vi "OT-PSD for stage.vi"() -> ()   [LabVIEW 2014]
uses:
  <vilib>/Analysis/2dsp.llb/Real FFT.vi
  <vilib>/Analysis/8numeric.llb/1D Numeric Integration.vi
  <vilib>/Utility/file.llb/Read From Spreadsheet File (DBL).vi
  <vilib>/Analysis/NI_AALPro.lvlib
  <vilib>/Analysis/NI_AALBase.lvlib
panel:
  out "variance":dbl format="%0.2f"
  out "standard deviation":dbl format="%0.2f"
  out "frequency":dbl[](array[numeric])
  out "Integrated freq":dbl[](array[numeric])
  out "df":dbl
  in  "sampling frequency (Hz)":i32
  in  "Tab Control":T1(tab)
  out "XY Graph":cluster{dbl[], "Filtered X":dbl[]}(graph)
  out "PSD 4":cluster{dbl[], dbl[]}(graph)
  out "PSD":cluster{dbl[], dbl[]}(graph)
  out "AutoPSD 2":cluster{dbl[], dbl[]}(graph)
  out "AutoPSD":cluster{dbl[], dbl[]}(graph)
  out "PSD 3":cluster{dbl[], dbl[]}(graph)
  out "PSD 2":cluster{dbl[], dbl[]}(graph)
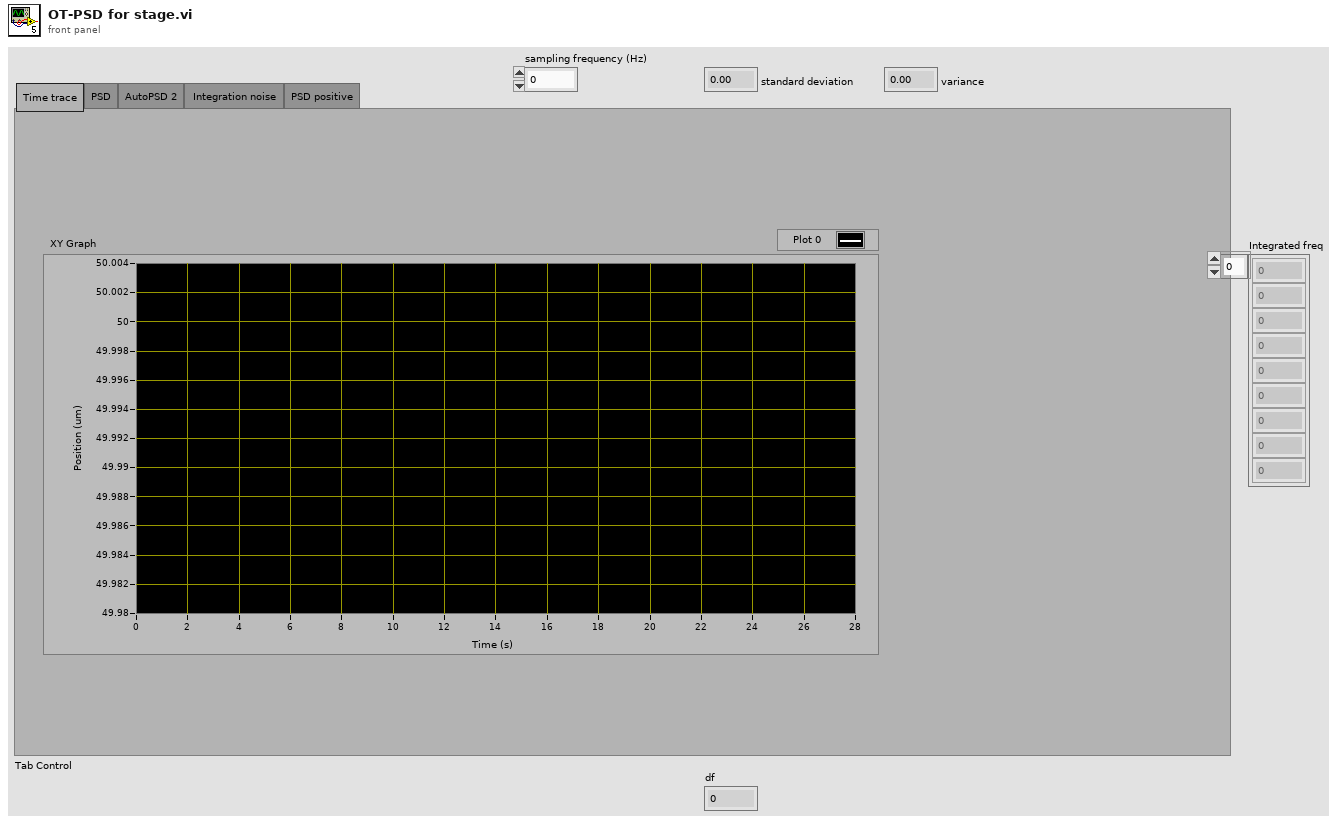
[diagram p1: front panel]
types:
  T1 = enum32{"Time trace", "PSD", "AutoPSD 2", "Integration noise ", "PSD positive"}
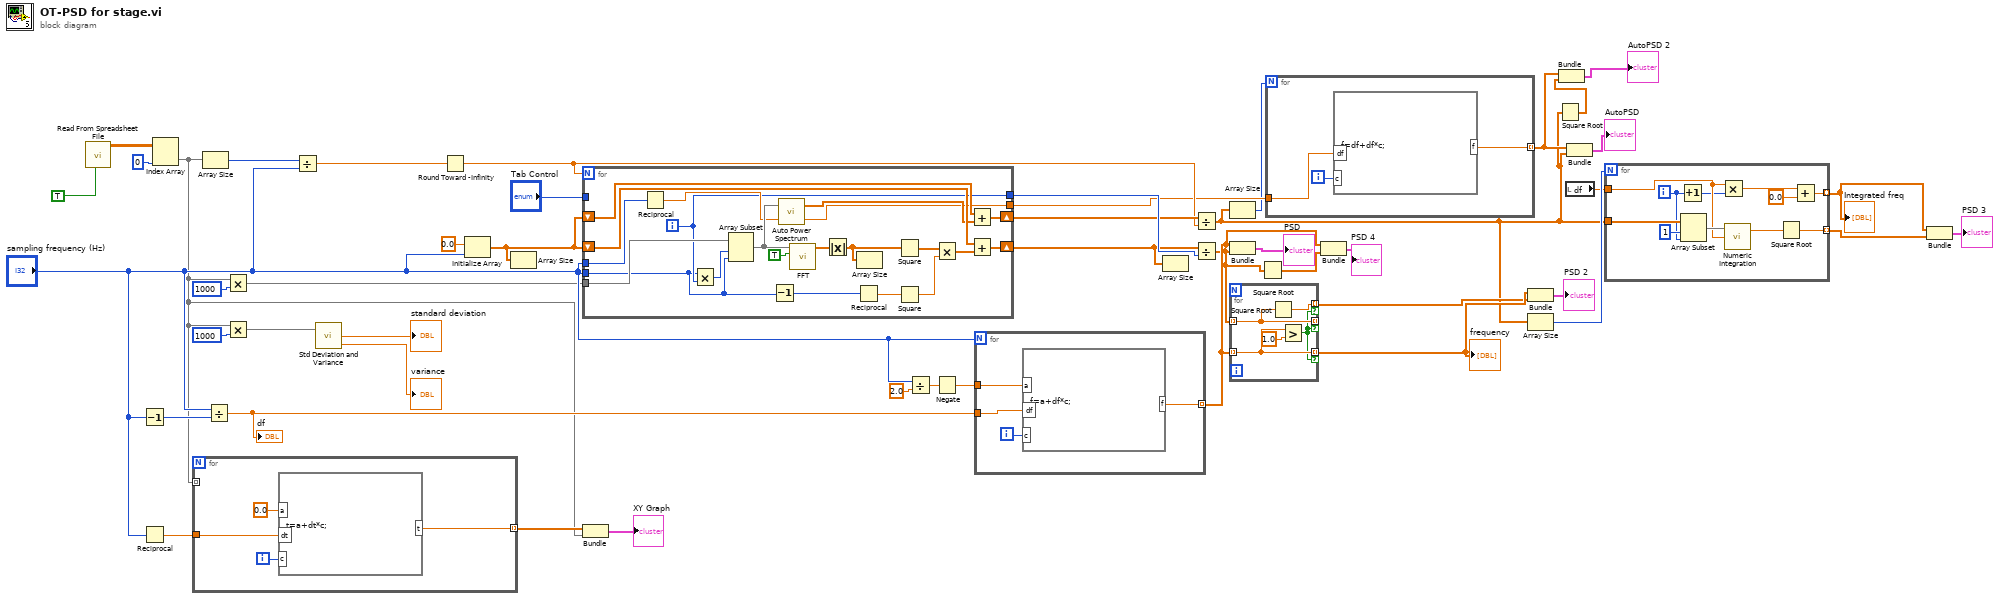
[diagram p0: block diagram]
diagram:
  n1 = call-poly <vilib>:"Read From Spreadsheet File.vi"("transpose (no:F)"=TRUE) -> ("all rows"=w48:dbl[][])  [unwired: 6 in, 4 out]
  n2 = Decrement(x="sampling frequency (Hz)") -> (x-1=w44:i32)
  n3 = Reciprocal(x="sampling frequency (Hz)") -> (1/x=w29:dbl)
  n4 = Index Array(array=w48, index (col)=0 ("disabled index (col)")) -> (element=w11:dbl[])  [unwired: 1 in]
  n5 = for {
    tunnel: w11 -> [_] mode=indexing
    tunnel: w29 -> [w50]
    tunnel: [w49] -> w32 mode=indexing
    i -> [w51]
    n6 = formula code="t=a+dt*c;"("a"=0.0 ("input variable"), "dt"=w50, "c"=w51) -> ("t"=w49:dbl)
  }
  n7 = Array Size(array=w11) -> (size(s)=w43:i32)
  n8 = Divide(x="sampling frequency (Hz)", y=w44) -> (x/y=w41:dbl)
  "df" <- w41
  n9 = Multiply(x=w11, y=1000) -> (x*y=w9:dbl[])
  n10 = Multiply(x=w11, y=1000) -> (x*y=w17:dbl[])
  n11 = Divide(x=w43, y="sampling frequency (Hz)") -> (x/y=w35:dbl)
  n12 = call <vilib>:"Std Deviation and Variance.vi"("X"=w17) -> ("standard deviation"=→"standard deviation":dbl, "variance"=→"variance":dbl)  [unwired: 1 in, 1 out]
  n13 = Round Toward -Infinity(1:w35) -> (0:w15:dbl)
  n14 = Initialize Array(0.0 ("element"), "sampling frequency (Hz)") -> (w36:dbl[])
  n15 = Array Size(array=w36) -> ()  [unwired: 1 out]
  n16 = for {
    N: w15 -> [_]
    tunnel: w9 -> [w73]
    tunnel: "sampling frequency (Hz)" -> [w54]
    shift-right: [w68] -> w37
    shift-left: w36 -> [w69]
    tunnel: "Tab Control" -> [_]
    tunnel: "sampling frequency (Hz)" -> [w65]
    shift-right: [w62] -> w16
    shift-left: w36 -> [w64]
    tunnel: [w61] -> w38
    tunnel: [w55] -> w14
    i -> [w61]
    n17 = Reciprocal(x=w65) -> (1/x=w66:dbl)
    n18 = Multiply(x=w54, y=w61) -> (x*y=w72:i32)
    n19 = Array Subset(array=w73, index=w72, length=w54) -> (w67:dbl[])
    n20 = Decrement(x=w54) -> (x-1=w53:i32)
    n21 = call <vilib>:"Auto Power Spectrum.vi"("dt"=w66, "Signal (V)"=w67) -> ("df"=w55:dbl, "Power Spectrum (V^2 rms)"=w63:dbl[])
    n22 = call-poly <vilib>:"FFT.vi"("shift?"=TRUE, "X"=w67) -> ("FFT {X}"=w70:cdb[])  [unwired: 8 in, 1 out]
    n23 = Absolute Value(x=w70) -> (abs(x)=w60:dbl[])
    n24 = Reciprocal(x=w53) -> (1/x=w58:dbl)
    n25 = Array Size(array=w60) -> ()  [unwired: 1 out]
    n26 = Square(x=w60) -> (x^2=w59:dbl[])
    n27 = Square(x=w58) -> (x^2=w57:dbl)
    n28 = Multiply(x=w59, y=w57) -> (x*y=w56:dbl[])
    n29 = Add(x=w64, y=w63) -> (x+y=w62:dbl[])
    n30 = Add(x=w69, y=w56) -> (x+y=w68:dbl[])
  }
  n31 = Bundle(w32, "all rows"=w11) -> (→"XY Graph":cluster{dbl[], "all rows":dbl[]})  [unwired: 1 in]
  n32 = Divide(x="sampling frequency (Hz)", y=2.0) -> (x/y=w45:dbl)
  n33 = Negate(x=w45) -> (-x=w42:dbl)
  n34 = for {
    N: "sampling frequency (Hz)" -> [_]
    tunnel: w42 -> [w77]
    tunnel: w41 -> [w76]
    tunnel: [w74] -> w8 mode=indexing
    i -> [w75]
    n35 = formula code="f=a+df*c;"("a"=w77, "df"=w76, "c"=w75) -> ("f"=w74:dbl)
  }
  n36 = Array Size(array=w37) -> ()  [unwired: 1 out]
  n37 = Divide(x=w16, y=w15) -> (x/y=w3:dbl[])
  n38 = Divide(x=w37, y=w38) -> (x/y=w7:dbl[])
  n39 = Array Size(array=w3) -> (size(s)=w13:i32)
  n40 = Bundle(w8, w7) -> (→"PSD":cluster{dbl[], dbl[]})  [unwired: 1 in]
  n41 = for {
    tunnel: [w80] -> w25 mode=indexing if=w78
    tunnel: w7 -> [w79] mode=indexing
    tunnel: w8 -> [w81] mode=indexing
    tunnel: [w81] -> w26 mode=indexing if=w78
    tunnel: [w79] -> _ mode=indexing if=w78
    n42 = Square Root(x=w79) -> (sqrt(x)=w80:dbl)
    n43 = Greater?(x=w81, y=1.0) -> (0:w78:bool)
  }
  "frequency" <- w26
  n44 = Square Root(x=w7) -> (sqrt(x)=w6:dbl[])
  n45 = for {
    N: w13 -> [_]
    tunnel: w14 -> [w85]
    tunnel: [w83] -> w4 mode=indexing
    i -> [w84]
    n46 = formula code="f=df+df*c;"("df"=w85, "c"=w84) -> ("f"=w83:dbl)
  }
  n47 = Bundle(w8, w6) -> (→"PSD 4":cluster{dbl[], dbl[]})  [unwired: 1 in]
  n48 = Bundle(w26, w25) -> (→"PSD 2":cluster{dbl[], dbl[]})  [unwired: 1 in]
  n49 = Array Size(array=w3) -> (size(s)=w28:i32)
  n50 = Square Root(x=w3) -> (sqrt(x)=w2:dbl[])
  n51 = Bundle(w4, w2) -> (→"AutoPSD 2":cluster{dbl[], dbl[]})  [unwired: 1 in]
  n52 = local read "df"() -> (w27:dbl)
  n53 = Bundle(w4, w3) -> (→"AutoPSD":cluster{dbl[], dbl[]})  [unwired: 1 in]
  n54 = for {
    N: w28 -> [_]
    tunnel: w3 -> [w96]
    tunnel: w27 -> [w93]
    tunnel: [w87] -> w22 mode=indexing
    tunnel: [w89] -> w23 mode=indexing
    i -> [w91]
    n55 = Increment(x=w91) -> (x+1=w92:i32)
    n56 = Array Subset(array=w96, index=1, length=w91) -> (w94:dbl[])
    n57 = Multiply(x=w93, y=w92) -> (x*y=w90:dbl)
    n58 = call-poly <vilib>:"Numeric Integration.vi"("dt"=w93, "Input Array"=w94) -> ("result"=w88:dbl)  [unwired: 1 in, 1 out]
    n59 = Square Root(x=w88) -> (sqrt(x)=w87:dbl)
    n60 = Add(x=w90, y=0.0) -> (x+y=w89:dbl)
  }
  "Integrated freq" <- w23
  n61 = Bundle(w23, w22) -> (→"PSD 3":cluster{dbl[], dbl[]})  [unwired: 1 in]
